vi "Pcre2SubstringByName8.vi"(8 "error in":errorcluster, 10 "Name":string, 11 "pMatchData":u64 format="%.0x") -> (0 "error out":errorcluster, 2 "Substring":string, 3 "pMatchData":u64 format="%.0x")   [LabVIEW 2021, in "libpcre2-8.lvlib"]
uses:
  libpcre2-8.lvlib
  Pcre2ErrorNull.vi
  Pcre2FnkCallError.vi
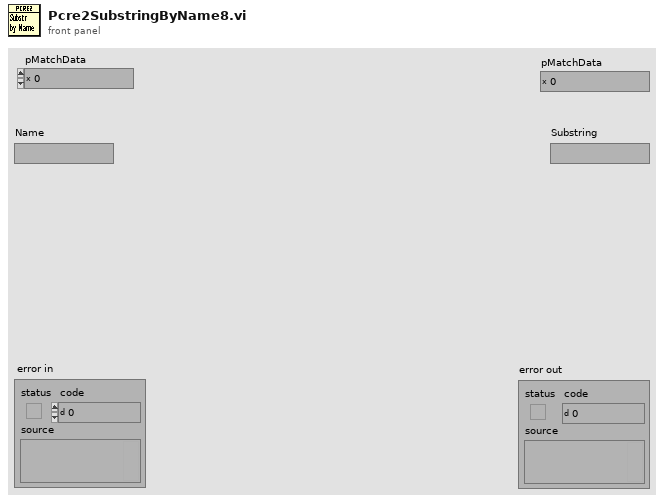
[diagram p1: front panel]
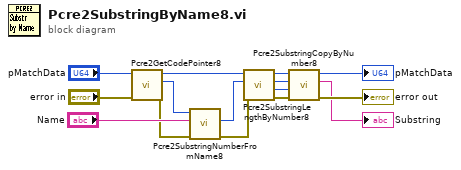
[diagram p0: block diagram]
diagram:
  n1 = call "Pcre2GetCodePointer8.vi"("error in"="error in", "pMatchData"="pMatchData") -> ("error out"=w8:errorcluster, "pCode"=w9:u64, "pMatchData"=w3:u64)  [unwired: 7 in]
  n2 = call "Pcre2SubstringNumberFromName8.vi"("error in"=w8, "Name"="Name", "pCode"=w9) -> ("error out"=w2:errorcluster, "Number"=w1:i32)  [unwired: 6 in, 1 out]
  n3 = call "Pcre2SubstringLengthByNumber8.vi"("error in"=w2, "Number"=w1, "pMatchData"=w3) -> ("error out"=w4:errorcluster, "Length"=w5:u64, "Number"=w6:i32, "pMatchData"=w7:u64)  [unwired: 5 in]
  n4 = call "Pcre2SubstringCopyByNumber8.vi"("error in"=w4, "Length"=w5, "Number"=w6, "pMatchData"=w7) -> ("error out"=→"error out":errorcluster, "Substring"=→"Substring":string, "pMatchData"=→"pMatchData":u64)  [unwired: 5 in]
